vi "Read Dots.vi"(8 "error in (no error)":errorcluster, 11 "Setting Database in":refnum<class "Setting Database.lvclass">) -> (0 "error out":errorcluster, 2 "Dots":refnum<class "Dot Settings.lvclass">[](array[class]), 3 "Setting Database out":refnum<class "Setting Database.lvclass">)   [LabVIEW 2019, in "Setting Database.lvclass"]
uses:
  Setting Database.lvclass
  Dot Settings/Dot Settings.lvclass
  Setting Database.lvclass/Setting Database.ctl
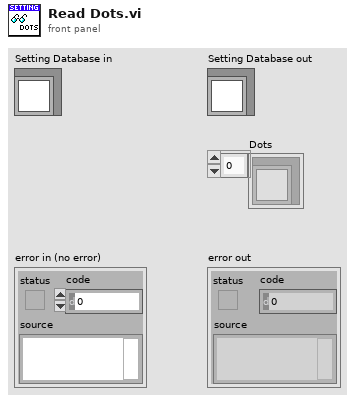
[diagram p1: front panel]
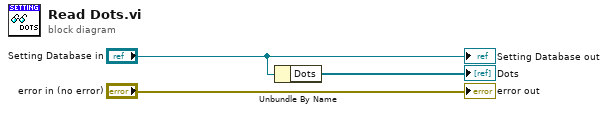
[diagram p0: block diagram]
diagram:
  n1 = Unbundle By Name("Setting Database in") -> ("Dots"=→"Dots":refnum<class "Dot Settings.lvclass">[])
  "error out" <- "error in (no error)"
  "Setting Database out" <- "Setting Database in"
